vi "Result.Generate Xlink Overall Result.vi"(10 "Measurements":T2[](array[typedef]) {"Status" items=["LOG", "PASS", "FAIL", "ERROR"]}, 11 "Result":T4) -> (2 "PASS":bool, 3 "Measurement":T1)   [LabVIEW 2019]
uses:
  Result XML/TestResult.Symptom.ctl
  Result XML/TestResult.Symptom.State.ctl
  Result.Measurement Item.ctl
  Result.Measurement and Attribute Item Status.ctl
  Result.Factory Logix XLink Adapter, Measurement Item.ctl
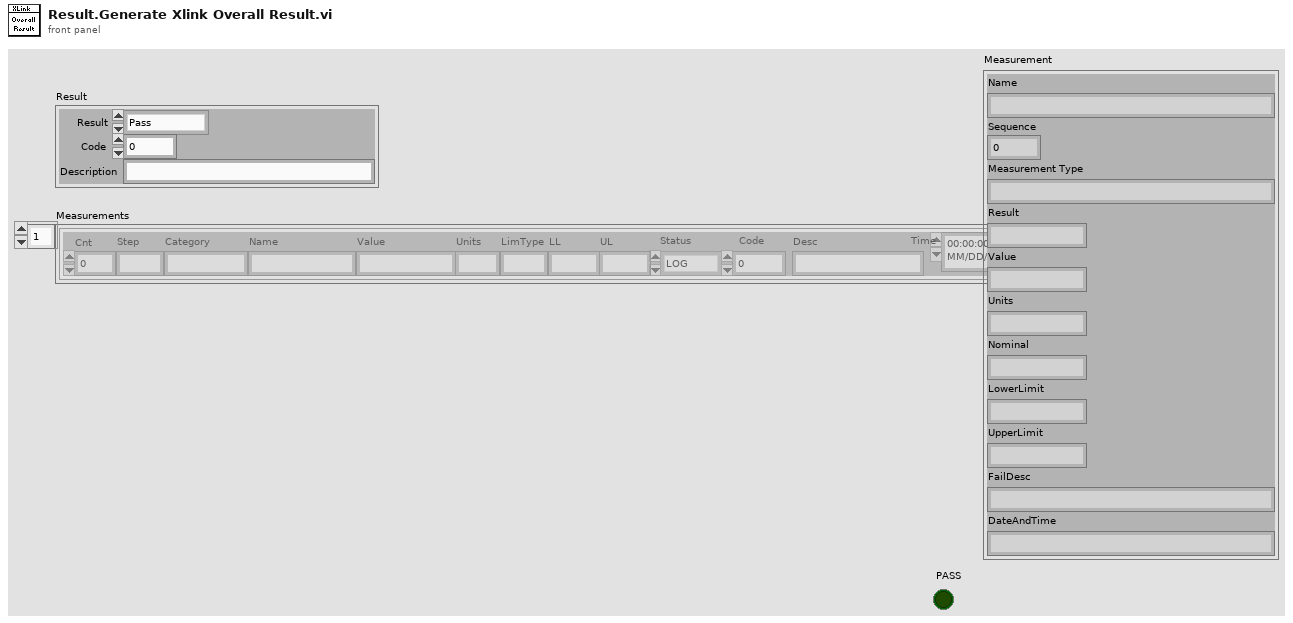
[diagram p1: front panel]
types:
  T1 = typedef "Result.Factory Logix XLink Adapter, Measurement Item.ctl" = cluster{"Name":string, "Sequence":i32, "Measurement Type":string, "Result":string, "Value":string, "Units":string, "Nominal":string, "LowerLimit":string, "UpperLimit":string, "FailDesc":string, "DateAndTime":string}
  T2 = typedef "Result.Measurement Item.ctl" = cluster{"Cnt":i32, "Step":string, "Category":string, "Name":string, "Value":string, "Units":string, "LimType":string, "LL":string, "UL":string, "Status":T3, "Code":i32, "Desc":string, "Time":timestamp}
  T3 = typedef "Result.Measurement and Attribute Item Status.ctl" = i32
  T4 = typedef "TestResult.Symptom.ctl" = cluster{"Result":T5, "Code":i32, "Description":string}
  T5 = typedef "TestResult.Symptom.State.ctl" = enum16{"Pass", "Fail", "Error", "Aborted", "Completed", "Logged"}
  T6 = cluster{"Pass":bool, "Code":string, "Name":string, "Meas":T1}
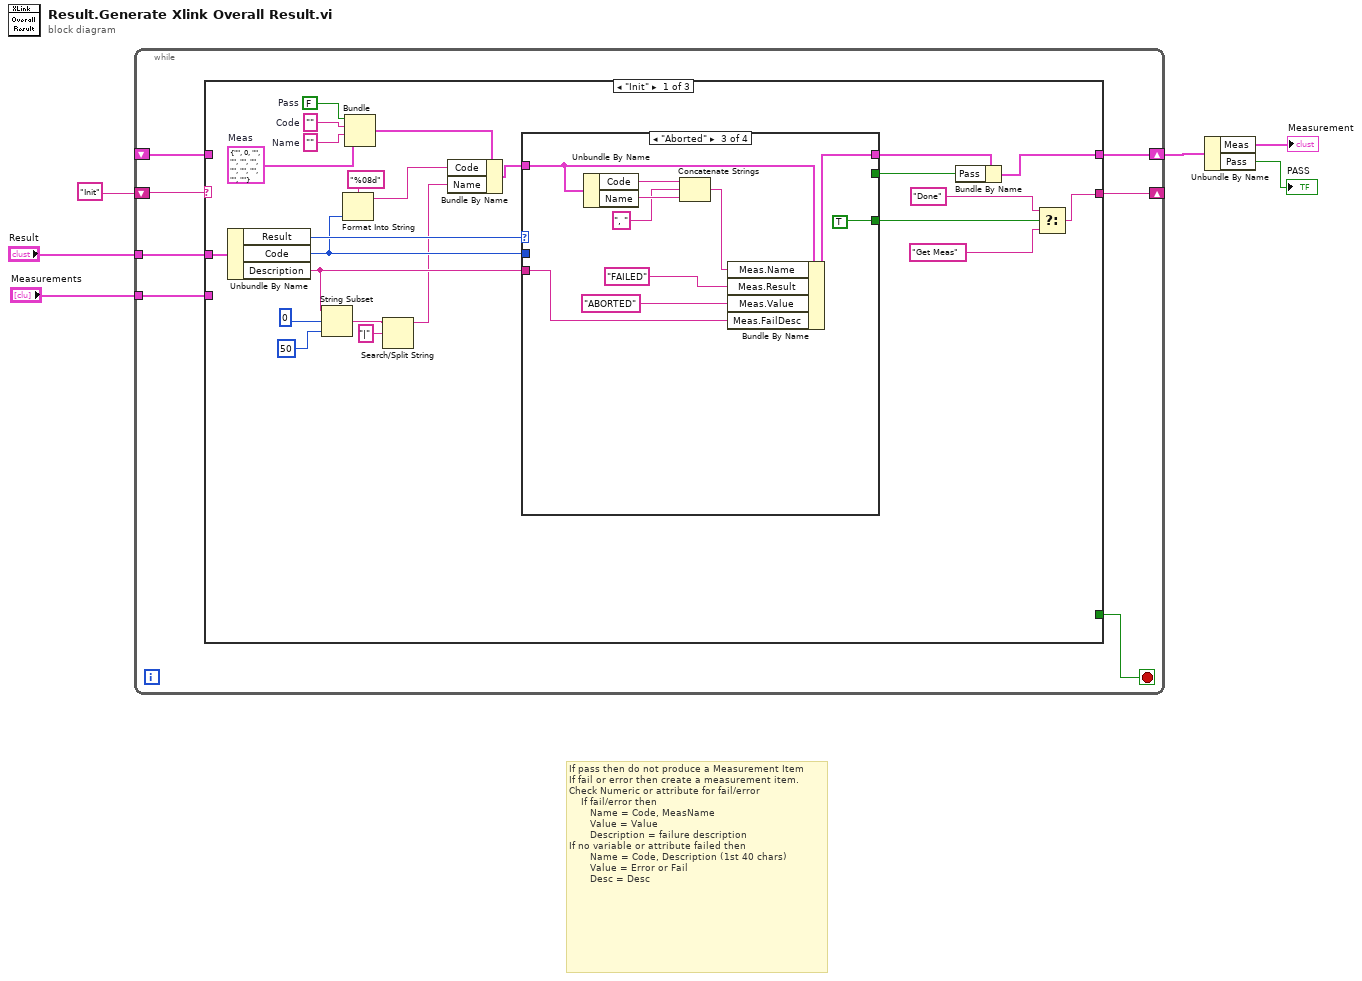
[diagram p0: block diagram]
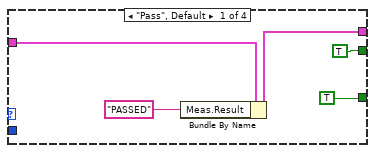
[diagram p2: hidden frame]
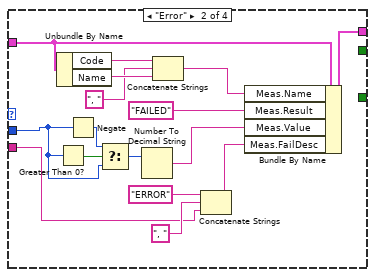
[diagram p3: hidden frame]
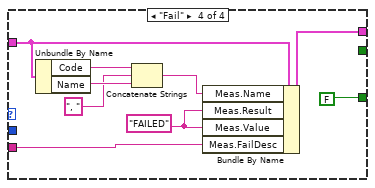
[diagram p4: hidden frame]
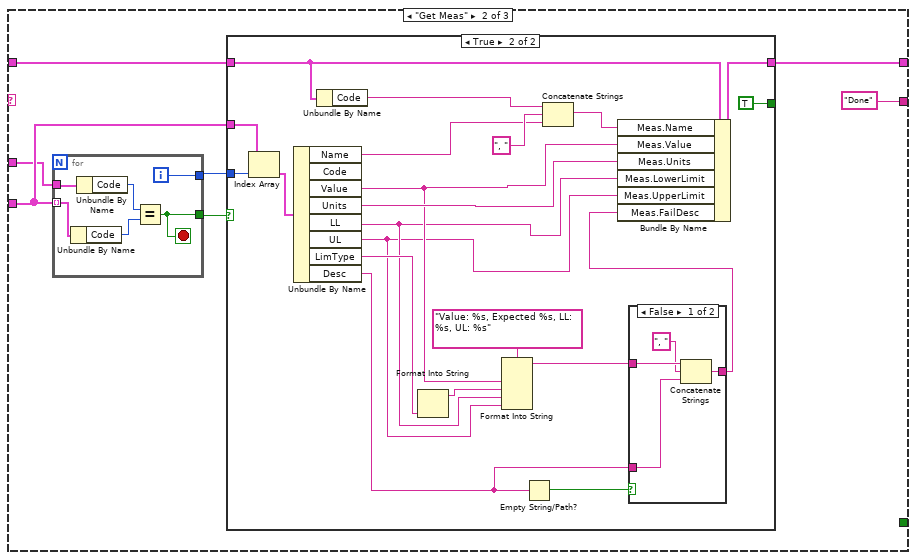
[diagram p5: hidden frame]
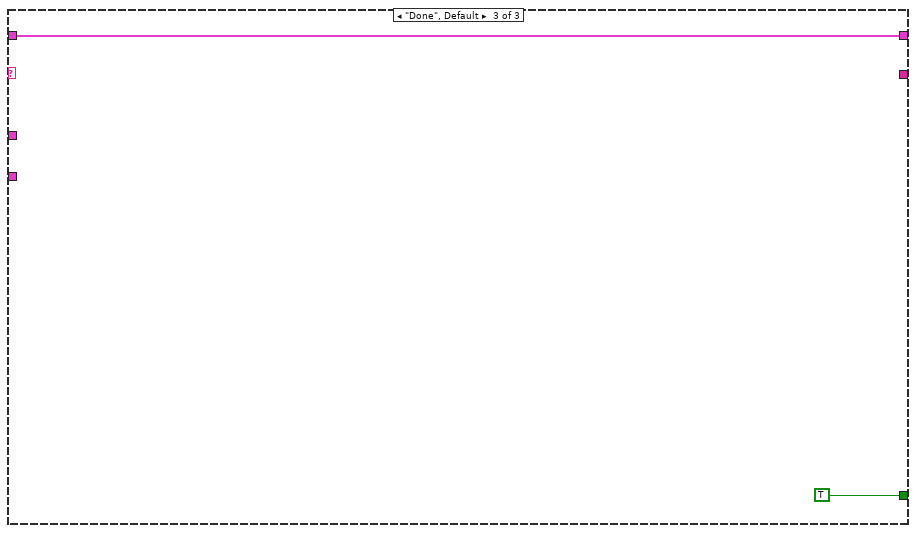
[diagram p8: hidden frame]
diagram:
  # "If pass then do not produce a Measurement Item\nIf fail or error then create a measurement item.\nCheck Numeric or attribute for fail/error\n    If fail/error then\n       Name = Code, MeasName\n       Value = Value\n       Description = failure description\nIf no variable or attribute failed then\n       Name = Code, Description (1st 40 chars)\n       Value = Error or Fail\n       Desc = Desc"
  n1 = while {
    shift-right: [w11] -> w3
    shift-left: _ -> [w13]
    shift-right: [w10] -> _
    shift-left: "Init" -> [w12]
    tunnel: "Result" -> [w8]
    tunnel: "Measurements" -> [w7]
    stop <- w9 stop-if-true
    n2 = case shown="\"Init\"" w12 {
      tunnel: w13 -> [_ w82 w118]
      tunnel: [w16 w81 w118] -> w11
      tunnel: [w35 "Done" _] -> w10
      tunnel: [_ _ TRUE] -> w9
      tunnel: w8 -> [w34 w79 _]
      tunnel: w7 -> [_ w83 _]
      frame "Init" {
        w18 = FALSE  # Pass
        w24 = ""  # Name
        w25 = ""  # Code
        w23 = T1 {"Name"="", "Sequence"=0, "Measurement Type"="", "Result"="", "Value"="", "Units"="", "Nominal"="", "LowerLimit"="", "UpperLimit"="", "FailDesc"="", "DateAndTime"=""}  # Meas
        n3 = Unbundle By Name(w34) -> ("Result"=w33:T5, "Code"=w26:i32, "Description"=w28:string)
        n4 = String Subset(string=w28, offset (0)=0, length (rest)=50 ("length (rest)")) -> (substring=w29:string)
        n5 = Format Into String(format string="%08d", w26) -> (resulting string=w20:string)  [unwired: 2 in, 1 out]
        n6 = Bundle("Pass"=w18, "Code"=w25, "Name"=w24, "Meas"=w23) -> (w22:T6)  [unwired: 1 in]
        n7 = Search/Split String(string=w29, search string/char (-)="|") -> (substring before match=w19:string)  [unwired: 1 in, 2 out]
        n8 = Bundle By Name(cluster=w22, "Code"=w20, "Name"=w19) -> (w21:T6)
        n9 = case shown="\"Aborted\"" w33 {
          tunnel: w21 -> [w41 w47 w61 w70]
          tunnel: w26 -> [_ w52 _ _]
          tunnel: w28 -> [_ w49 w65 w74]
          tunnel: [w40 w58 w68 w77] -> w17
          tunnel: [TRUE _ TRUE FALSE] -> w15
          tunnel: [TRUE _ _ _] -> w14
          frame "Pass", Default {
            n10 = Bundle By Name(cluster=w41, "Meas.Result"="PASSED" ("Result")) -> (w40:T6)
          }
          frame "Error" {
            n11 = Unbundle By Name(w47) -> ("Code"=w46:string, "Name"=w45:string)
            n12 = Greater Than 0?(x=w52) -> (x > 0?=w54:bool)
            n13 = Negate(x=w52) -> (-x=w55:i32)
            n14 = Select(t=w55, s=w54, f=w52) -> (s? t:f=w51:i32)
            n15 = Number To Decimal String(number=w51) -> (decimal integer string=w48:string)  [unwired: 1 in]
            n16 = Concatenate Strings(w46, ", ", w45) -> (w43:string)
            n17 = Concatenate Strings("ERROR" ("Result"), ", ", w49) -> (w56:string)
            n18 = Bundle By Name(cluster=w47, "Meas.Name"=w43, "Meas.Result"="FAILED" ("Result"), "Meas.Value"=w48, "Meas.FailDesc"=w56) -> (w58:T6)
          }
          frame "Aborted" {
            n19 = Unbundle By Name(w61) -> ("Code"=w64:string, "Name"=w63:string)
            n20 = Concatenate Strings(w64, ", ", w63) -> (w60:string)
            n21 = Bundle By Name(cluster=w61, "Meas.Name"=w60, "Meas.Result"="FAILED" ("Result"), "Meas.Value"="ABORTED" ("Result"), "Meas.FailDesc"=w65) -> (w68:T6)
          }
          frame "Fail" {
            w75 = "FAILED" ("Result")
            n22 = Unbundle By Name(w70) -> ("Code"=w73:string, "Name"=w72:string)
            n23 = Concatenate Strings(w73, ", ", w72) -> (w69:string)
            n24 = Bundle By Name(cluster=w70, "Meas.Name"=w69, "Meas.Result"=w75, "Meas.Value"=w75, "Meas.FailDesc"=w74) -> (w77:T6)
          }
        }
        n25 = Bundle By Name(cluster=w17, "Pass"=w14) -> (w16:T6)
        n26 = Select(t="Done", s=w15, f="Get Meas") -> (s? t:f=w35:string)
      }
      frame "Get Meas" {
        n27 = for {
          tunnel: w83 -> [w117] mode=indexing
          tunnel: [w116] -> w80
          tunnel: [w115] -> w84
          tunnel: w79 -> [w113]
          i -> [w115]
          stop <- w116 stop-if-true
          n28 = Unbundle By Name(w117) -> ("Code"=w114:i32)
          n29 = Unbundle By Name(w113) -> ("Code"=w112:i32)
          n30 = Equal?(x=w112, y=w114) -> (x = y?=w116:bool)
        }
        n31 = case shown="True" w80 {
          tunnel: w84 -> [_ w106]
          tunnel: w83 -> [_ w105]
          tunnel: w82 -> [w85 w90]
          tunnel: [w85 w102] -> w81
          tunnel: [_ TRUE] -> _
          frame False {
          }
          frame True {
            n32 = Index Array(array=w105, index=w106) -> (element=w104:T2)
            n33 = Unbundle By Name(w104) -> ("Name"=w91:string, "Value"=w88:string, "Units"=w100:string, "LL"=w87:string, "UL"=w86:string, "LimType"=w96:string, "Desc"=w95:string)  [unwired: 1 out]
            n34 = Unbundle By Name(w90) -> ("Code"=w89:string)
            n35 = Format Into String(w96) -> (resulting string=w97:string)  [unwired: 3 in, 1 out]
            n36 = Format Into String(format string="Value: %s, Expected %s, LL: %s, UL: %s", w88, w97, w87, w86) -> (resulting string=w98:string)  [unwired: 2 in, 1 out]
            n37 = Empty String/Path?(string/path=w95) -> (empty?=w94:bool)
            n38 = Concatenate Strings(w89, ", ", w91) -> (w101:string)
            n39 = case shown="False" w94 {
              tunnel: w98 -> [w110 w111]
              tunnel: w95 -> [w109 _]
              tunnel: [w107 w111] -> w93
              frame False {
                n40 = Concatenate Strings(w110, ", ", w109) -> (w107:string)
              }
              frame True {
              }
            }
            n41 = Bundle By Name(cluster=w90, "Meas.Name"=w101, "Meas.Value"=w88, "Meas.Units"=w100, "Meas.LowerLimit"=w87, "Meas.UpperLimit"=w86, "Meas.FailDesc"=w93) -> (w102:T6)
          }
        }
      }
      frame "Done", Default {
      }
    }
  }
  n42 = Unbundle By Name(w3) -> ("Meas"=→"Measurement":T1, "Pass"=→"PASS":bool)
